vi "Verify - Check Poly Fields.vi"(8 "error in (no error)":errorcluster, 9 "InstanceInfo":T1={"VIPath"=path "C:/Projects/GitHub/data-record-ad-internal/Data Types/ADAS Generic/Read.vi", "Menu Name"="Generic", "Selector Name"="Generic"}, 10 "Poly Ref":refnum<vi>, 11 "Poly Map Set in":T2) -> (0 "error out":errorcluster, 1 "Error?":string)   [LabVIEW 2020]
uses:
  _td_map_PolyInstanceInfo.ctl
  _td_cluster_InstanceInfo.ctl
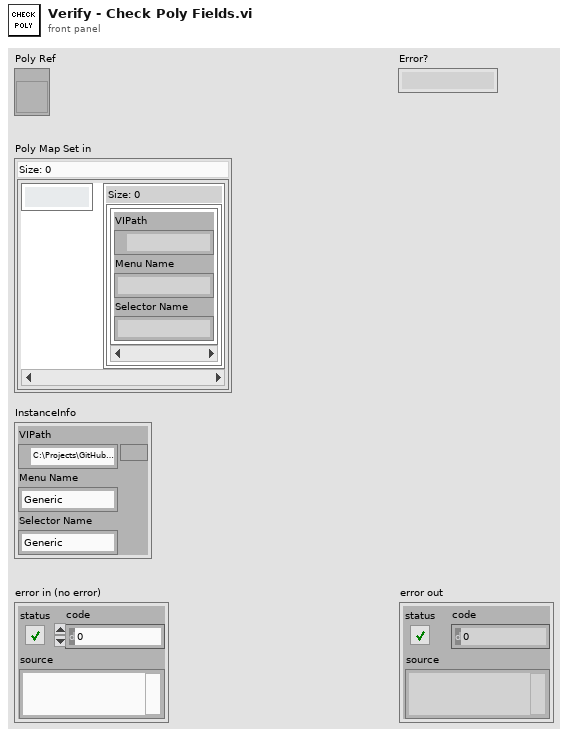
[diagram p1: front panel]
types:
  T1 = typedef "_td_cluster_InstanceInfo.ctl" = cluster{"VIPath":path, "Menu Name":string, "Selector Name":string}
  T2 = typedef "_td_map_PolyInstanceInfo.ctl" = map{string, set{T1}}
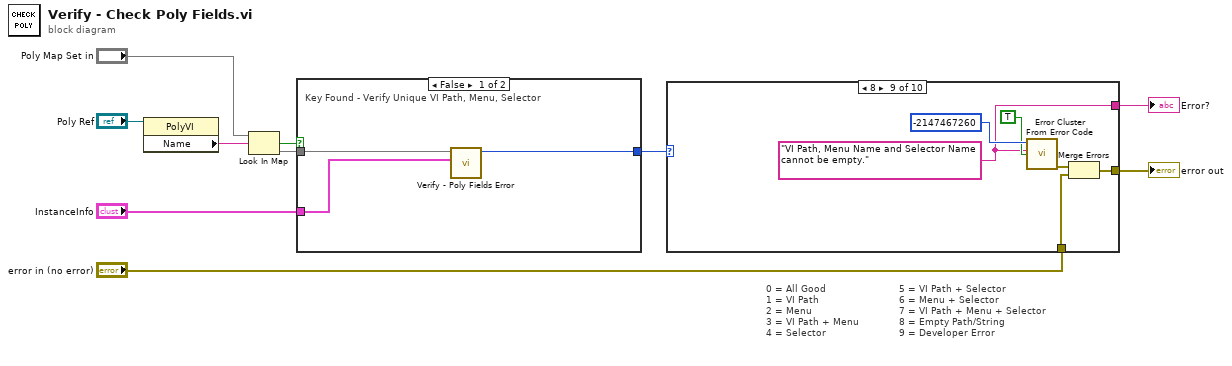
[diagram p0: block diagram]
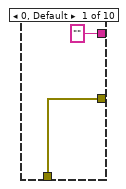
[diagram p2: hidden frame]
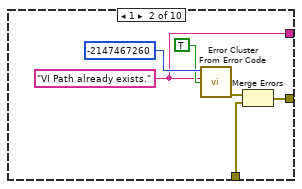
[diagram p3: hidden frame]
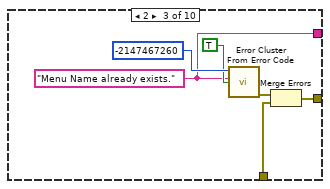
[diagram p4: hidden frame]
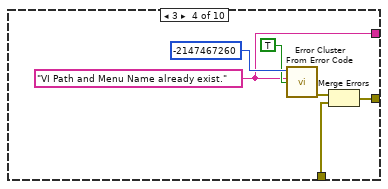
[diagram p5: hidden frame]
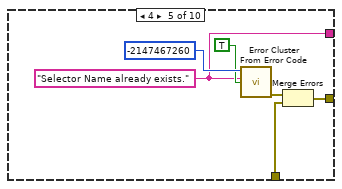
[diagram p6: hidden frame]
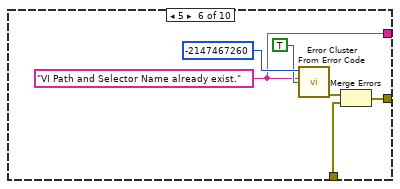
[diagram p7: hidden frame]
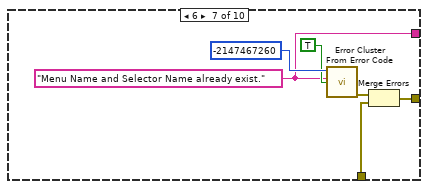
[diagram p8: hidden frame]
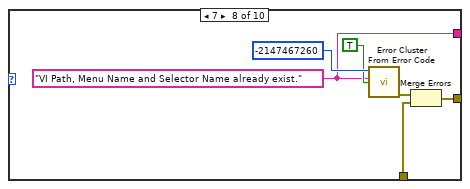
[diagram p9: hidden frame]
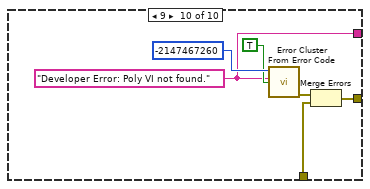
[diagram p10: hidden frame]
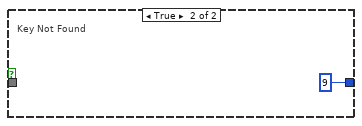
[diagram p11: hidden frame]
diagram:
  # "5 = VI Path + Selector \n6 = Menu + Selector \n7 = VI Path + Menu + Selector\n8 = Empty Path/String\n9 = Developer Error"
  # "0 = All Good\n1 = VI Path\n2 = Menu \n3 = VI Path + Menu \n4 = Selector"
  n1 = property class="PolyVI"(reference="Poly Ref") -> ("Name"=w5:string)  [unwired: 1 in, 2 out]
  n2 = Look In Map(map="Poly Map Set in", key=w5) -> (key not found?=w2:bool, value=w3:set{T1})  [unwired: 1 in]
  n3 = case shown="False" w2 {
    tunnel: w3 -> [w13 _]
    tunnel: [w11 u32 9] -> w1
    tunnel: "InstanceInfo" -> [w12 _]
    frame False {
      # "Key Found - Verify Unique VI Path, Menu, Selector"
      n4 = call "Verify - Poly Fields Error.vi"("Instance Info"=w12, "Poly Set"=w13) -> ("Error"=w11:u32)  [unwired: 9 in]
    }
    frame True {
      # "Key Not Found"
    }
  }
  n5 = case shown="8" w1 {
    tunnel: "error in (no error)" -> [w16 w19 w25 w31 w37 w43 w49 w55 w61 w67]
    tunnel: [w16 w18 w24 w30 w36 w42 w48 w54 w60 w66] -> w8
    tunnel: ["" w17 w23 w29 w35 w41 w47 w53 w59 w65] -> w7
    frame 0, Default {
    }
    frame 1 {
      w17 = "VI Path already exists."
      n6 = call <vilib>:"Error Cluster From Error Code.vi"("show call chain? (False)"=TRUE, "error message (\"\")"=w17, "error code (0)"=-2147467260) -> ("error out"=w20:errorcluster)  [unwired: 6 in]
      n7 = Merge Errors(w20, w19) -> (w18:errorcluster)
    }
    frame 2 {
      w23 = "Menu Name already exists."
      n8 = call <vilib>:"Error Cluster From Error Code.vi"("show call chain? (False)"=TRUE, "error message (\"\")"=w23, "error code (0)"=-2147467260) -> ("error out"=w26:errorcluster)  [unwired: 6 in]
      n9 = Merge Errors(w26, w25) -> (w24:errorcluster)
    }
    frame 3 {
      w29 = "VI Path and Menu Name already exist."
      n10 = call <vilib>:"Error Cluster From Error Code.vi"("show call chain? (False)"=TRUE, "error message (\"\")"=w29, "error code (0)"=-2147467260) -> ("error out"=w32:errorcluster)  [unwired: 6 in]
      n11 = Merge Errors(w32, w31) -> (w30:errorcluster)
    }
    frame 4 {
      w35 = "Selector Name already exists."
      n12 = call <vilib>:"Error Cluster From Error Code.vi"("show call chain? (False)"=TRUE, "error message (\"\")"=w35, "error code (0)"=-2147467260) -> ("error out"=w38:errorcluster)  [unwired: 6 in]
      n13 = Merge Errors(w38, w37) -> (w36:errorcluster)
    }
    frame 5 {
      w41 = "VI Path and Selector Name already exist."
      n14 = call <vilib>:"Error Cluster From Error Code.vi"("show call chain? (False)"=TRUE, "error message (\"\")"=w41, "error code (0)"=-2147467260) -> ("error out"=w44:errorcluster)  [unwired: 6 in]
      n15 = Merge Errors(w44, w43) -> (w42:errorcluster)
    }
    frame 6 {
      w47 = "Menu Name and Selector Name already exist."
      n16 = call <vilib>:"Error Cluster From Error Code.vi"("show call chain? (False)"=TRUE, "error message (\"\")"=w47, "error code (0)"=-2147467260) -> ("error out"=w50:errorcluster)  [unwired: 6 in]
      n17 = Merge Errors(w50, w49) -> (w48:errorcluster)
    }
    frame 7 {
      w53 = "VI Path, Menu Name and Selector Name already exist."
      n18 = call <vilib>:"Error Cluster From Error Code.vi"("show call chain? (False)"=TRUE, "error message (\"\")"=w53, "error code (0)"=-2147467260) -> ("error out"=w56:errorcluster)  [unwired: 6 in]
      n19 = Merge Errors(w56, w55) -> (w54:errorcluster)
    }
    frame 8 {
      w59 = "VI Path, Menu Name and Selector Name cannot be empty."
      n20 = call <vilib>:"Error Cluster From Error Code.vi"("show call chain? (False)"=TRUE, "error message (\"\")"=w59, "error code (0)"=-2147467260) -> ("error out"=w62:errorcluster)  [unwired: 6 in]
      n21 = Merge Errors(w62, w61) -> (w60:errorcluster)
    }
    frame 9 {
      w65 = "Developer Error: Poly VI not found."
      n22 = call <vilib>:"Error Cluster From Error Code.vi"("show call chain? (False)"=TRUE, "error message (\"\")"=w65, "error code (0)"=-2147467260) -> ("error out"=w68:errorcluster)  [unwired: 6 in]
      n23 = Merge Errors(w68, w67) -> (w66:errorcluster)
    }
  }
  "error out" <- w8
  "Error?" <- w7
